vi "Teleop.vi"(10 "Match Info":T1={"Autonomous Elapsed Seconds"=0.0, "TeleOp Elapsed Seconds"=0.0, "Disabled Elapsed Seconds"=0.0, "Visited Autonomous"=FALSE, "Visited TeleOp"=FALSE, "Visited Disabled"=FALSE, "Autonomous Settings"={"Autonomous Style"=enum."Independent", "VI Refnum"=refnum}}, 11 "Call Context":T2) -> ()   [LabVIEW 2012]
doc: "This VI is called for each TeleOp packet received from the DS where the robot is not disabled. It is often used to read from the joysticks and update I/O or to update setpoints for timed control loops. It should complete and return within 20 milliseconds or it may miss DS packets."
uses:
  <vilib>/Rock Robotics/WPI/DriverStation/WPI_DriverStationDerivedRobotMode.ctl
  <vilib>/Rock Robotics/WPI/DriverStation/WPI_DriverStationMatch Info.ctl
  Robot Global Data.vi
  <vilib>/Rock Robotics/Network Tables/SD Write Boolean.vi
  <vilib>/Rock Robotics/WPI/Joystick/WPI_JoystickGetSetRefNum.vi
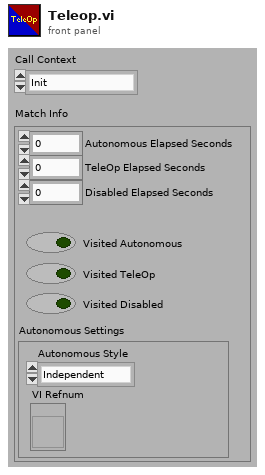
[diagram p1: front panel]
types:
  T1 = typedef "WPI_DriverStationMatch Info.ctl" = cluster{"Autonomous Elapsed Seconds":dbl, "TeleOp Elapsed Seconds":dbl, "Disabled Elapsed Seconds":dbl, "Visited Autonomous":bool, "Visited TeleOp":bool, "Visited Disabled":bool, "Autonomous Settings":cluster{"Autonomous Style":enum16{"Iterative", "Independent"}, "VI Refnum":refnum<vi>}}
  T2 = typedef "WPI_DriverStationDerivedRobotMode.ctl" = enum16{"Init", "Execute", "Stop"}
  T3 = enum16{"Off", "Close Pyramid 3pt", "Far Pyramid 3pt", "Feeder Shot", "UD Far 3pt Shot"}
  T4 = typedef "WPI_JoystickDevRef.ctl" = cluster{"Device":T5}
  T5 = typedef "WPI_JoystickDeviceEnum.ctl" = enum16{"USB 1", "USB 2", "USB 3", "USB 4", "Kinect 1", "Kinect 2"}
  T6 = typedef "WPI_JoystickButtonState.ctl" = cluster{"Button 1":bool, "Button 2":bool, "Button 3":bool, "Button 4":bool, "Button 5":bool, "Button 6":bool, "Button 7":bool, "Button 8":bool, "Button 9":bool, "Button 10":bool, "Button 11":bool, "Button 12":bool}
  T7 = cluster{"axis 1 (x)":dbl, "axis 2 (y)":dbl, "axis 3 (throttle)":dbl, "axis 4":dbl, "axis 5":dbl, "axis 6":dbl}
  T8 = enum16{"Close 3pt Shot", "Far 3pt Shot", "Feeding"}
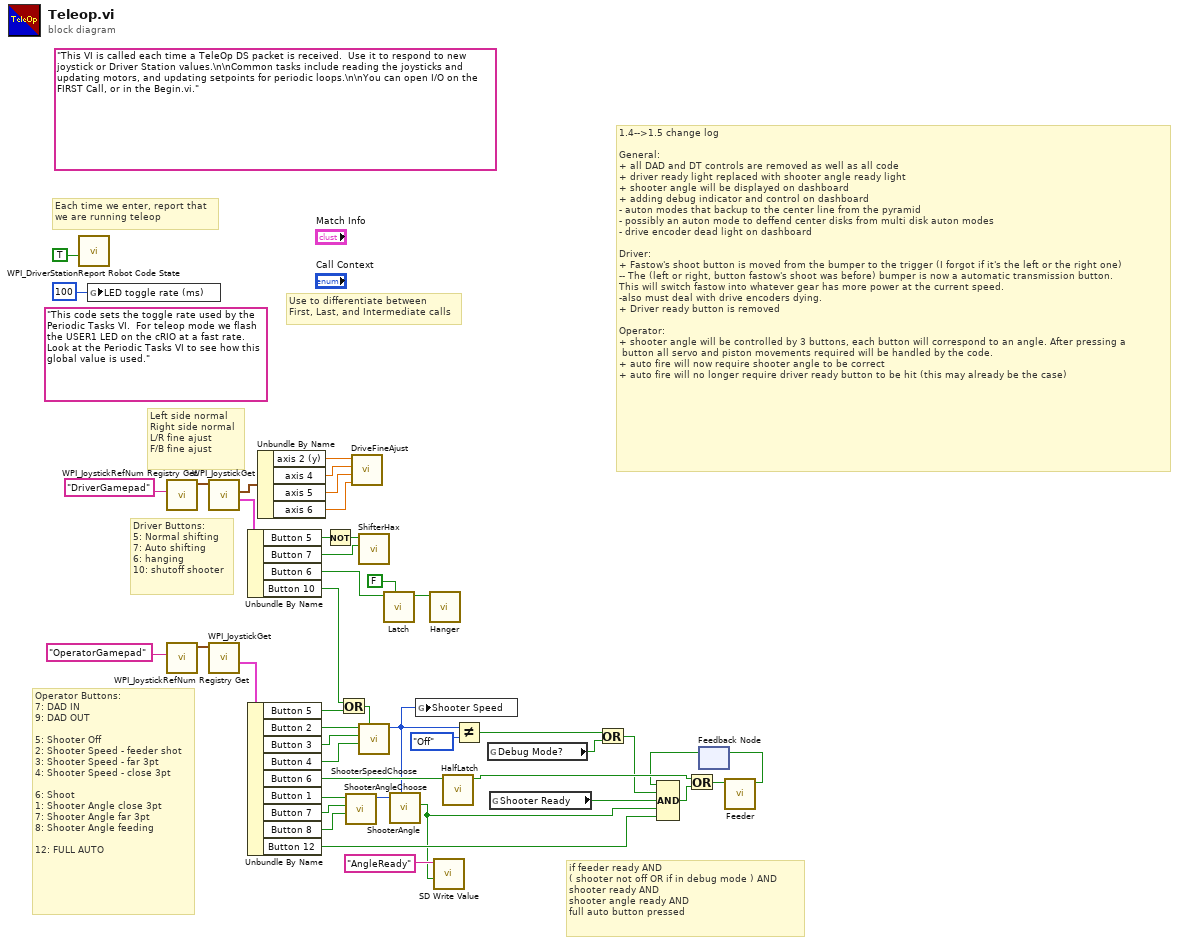
[diagram p0: block diagram]
diagram:
  (unwired) "This code sets the toggle rate used by the Periodic Tasks VI.  For teleop mode we flash the USER1 LED on the cRIO at a fast rate.  Look at the Periodic Tasks VI to see how this global value is used."
  (unwired) "This VI is called each time a TeleOp DS packet is received.  Use it to respond to new joystick or Driver Station values.\n\nCommon tasks include reading the joysticks and updating motors, and updating setpoints for periodic loops.\n\nYou can open I/O on the FIRST Call, or in the Begin.vi."
  # "1.4-->1.5 change log\n\nGeneral:\n+ all DAD and DT controls are removed as well as all code\n+ driver ready light replaced with shooter angle ready light\n+ shooter angle will be displayed on dashboard\n+ adding debug indicator and control on dashboard\n- auton modes that backup to the center line from the pyramid\n- possibly an auton mode to deffend center disks from multi disk auton modes\n- drive encoder dead light on dashboard\n\nDriver:\n+ Fastow's shoot button is moved from the bumper to the trigger (I forgot if it's the left or the right one)\n-- The (left or right, button fastow's shoot was before) bumper is now a automatic transmission button. \nThis will switch fastow into whatever gear has more power at the current speed.\n-also must deal with drive encoders dying.\n+ Driver ready button is removed\n\nOperator:\n+ shooter angle will be controlled by 3 buttons, each button will correspond to an angle. After pressing a\n button all servo and piston movements required will be handled by the code.\n+ auto fire will now require shooter angle to be correct\n+ auto fire will no longer require driver ready button to be hit (this may already be the case)"
  # "Left side normal\nRight side normal\nL/R fine ajust\nF/B fine ajust"
  # "if feeder ready AND\n( shooter not off OR if in debug mode ) AND\nshooter ready AND\nshooter angle ready AND\nfull auto button pressed"
  # "Driver Buttons:\n5: Normal shifting\n7: Auto shifting\n6: hanging\n10: shutoff shooter"
  # "Operator Buttons:\n7: DAD IN\n9: DAD OUT\n\n5: Shooter Off\n2: Shooter Speed - feeder shot\n3: Shooter Speed - far 3pt\n4: Shooter Speed - close 3pt\n\n6: Shoot\n1: Shooter Angle close 3pt\n7: Shooter Angle far 3pt\n8: Shooter Angle feeding\n\n12: FULL AUTO"
  # "Each time we enter, report that\nwe are running teleop"
  # "Use to differentiate between\nFirst, Last, and Intermediate calls"
  n1 = call <vilib>:"WPI_DriverStationReport Robot Code State.vi"("TeleOp"=TRUE ("Autonomous")) -> ()  [unwired: 10 in, 1 out]
  n2 = global write "Robot Global Data.vi" "LED toggle rate (ms)"(u32 100 ("LED ms toggle rate")) -> ()
  n3 = call <vilib>:"WPI_JoystickRefNum Registry Get.vi"("refnum name"="DriverGamepad") -> ("JoystickDevRef"=w44:T4)  [unwired: 1 in, 9 out]
  n4 = call <vilib>:"WPI_JoystickRefNum Registry Get.vi"("refnum name"="OperatorGamepad") -> ("JoystickDevRef"=w39:T4)  [unwired: 1 in, 9 out]
  n5 = call <vilib>:"WPI_JoystickGet.vi"("JoystickDevRef"=w44) -> ("Buttons"=w40:T6, "Axes"=w41:T7)  [unwired: 1 in, 4 out]
  n6 = call <vilib>:"WPI_JoystickGet.vi"("JoystickDevRef"=w39) -> ("Buttons"=w38:T6)  [unwired: 1 in, 5 out]
  n7 = Unbundle By Name(w40) -> ("Button 5"=w20:bool, "Button 7"=w7:bool, "Button 6"=w6:bool, "Button 10"=w5:bool)
  n8 = Unbundle By Name(w38) -> ("Button 5"=w34:bool, "Button 2"=w33:bool, "Button 3"=w32:bool, "Button 4"=w31:bool, "Button 6"=w19:bool, "Button 1"=w10:bool, "Button 7"=w9:bool, "Button 8"=w8:bool, "Button 12"=w12:bool)
  n9 = Unbundle By Name(w41) -> ("axis 2 (y)"=w23:dbl, "axis 4"=w22:dbl, "axis 5"=w25:dbl, "axis 6"=w24:dbl)
  n10 = Not(x=w20) -> (.not. x?=w21:bool)
  n11 = Or(x=w5, y=w34) -> (x .or. y?=w30:bool)
  n12 = call "ShooterAngleChoose.vi"("Feeding Button"=w8, "Far 3pt Buton"=w9, "Close 3pt Button"=w10) -> ("Target Shooter Angle"=w11:T8)  [unwired: 8 in]
  n13 = call "DriveFineAjust.vi"("Fine Ajust F/B"=w24, "Fine Ajust L/R"=w25, "Right Side Normal"=w22, "Left Side Normal"=w23) -> ()  [unwired: 8 in]
  n14 = call "ShifterHax.vi"("Automatic Shifting"=w7, "Manual Shift Low"=w21) -> ()  [unwired: 10 in]
  n15 = call "ShooterSpeedChoose.vi"("Shooter OFF"=w30, "Close 3pt Shot Button"=w31, "Far 3pt Shot Button"=w32, "Feedershot Button"=w33) -> ("Shooter Speed"=w13:T3)  [unwired: 7 in]
  n16 = call "Latch.vi"("Default Value (false)"=FALSE, "Latch In"=w6) -> ("Latch Out"=w37:bool)  [unwired: 9 in]
  n17 = call "ShooterAngle.vi"("Shooter Speed"=w13, "Target Shooter Angle"=w11) -> ("Shooter Angle Done"=w1:bool)  [unwired: 8 in, 1 out]
  n18 = global write "Robot Global Data.vi" "Shooter Speed"(w13) -> ()
  n19 = call "Hanger.vi"("Hanger Up"=w37) -> ()  [unwired: 10 in, 1 out]
  n20 = call-poly <vilib>:"SD Write Value.vi"("Boolean"=w1, "Name"="AngleReady") -> ()  [unwired: 8 in, 2 out]
  n21 = call "HalfLatch.vi"("Input"=w19) -> ("Output"=w18:bool)  [unwired: 10 in]
  n22 = Not Equal?(x=w13, y=T3."Off" ("Shooter Speed")) -> (x != y?=w16:bool)
  n23 = global read "Robot Global Data.vi" "Debug Mode?"() -> (w15:bool)
  n24 = global read "Robot Global Data.vi" "Shooter Ready"() -> (w2:bool)
  n25 = Or(x=w16, y=w15) -> (x .or. y?=w3:bool)
  n26 = feedback #1() -> (w4:bool)  [unwired: 1 in]
  n27 = Compound Arithmetic op=AND(w4, w3, w2, w1, w12) -> (w28:bool)
  n28 = Or(x=w18, y=w28) -> (x .or. y?=w29:bool)
  n29 = call "Feeder.vi"("SHOOT Button"=w29) -> ("Ready To Shoot?"=w27:bool)  [unwired: 10 in]
  n30 = feedback-in #1(w27) -> ()
